vi "Disconnect.vi"(8 "error in (no error)":errorcluster, 11 "Network Stream in":refnum<class "Network Stream.lvclass">) -> (0 "error out":errorcluster, 3 "Network Stream out":refnum<class "Network Stream.lvclass">)   [LabVIEW 2020, in "Network Stream.lvclass"]
uses:
  Network Stream.lvclass
  Network Stream.lvclass/Network Stream.ctl
  <vilib>/dex/Flush And Wait Empty Condition.ctl
  <resource>/objmgr/ni.dex.rc
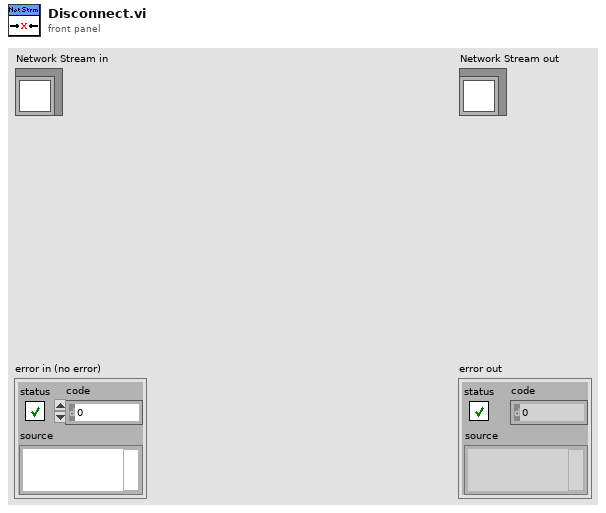
[diagram p1: front panel]
types:
  T1 = typedef "Flush And Wait Empty Condition.ctl" = u8
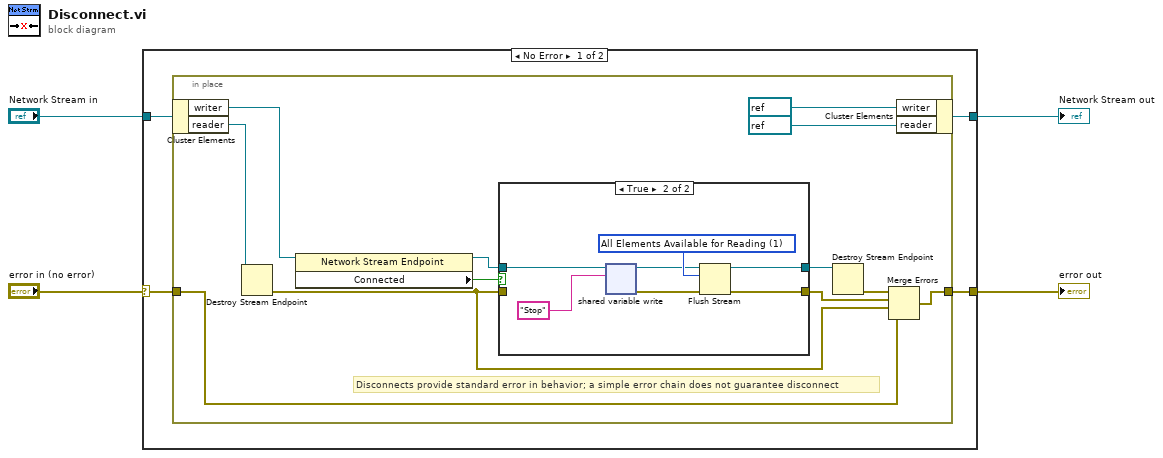
[diagram p0: block diagram]
diagram:
  n1 = case shown="No Error" "error in (no error)" {
    selector: "error in (no error)" -> [w8 w30]
    tunnel: [w5 w30] -> w1
    tunnel: [w7 w29] -> w3
    tunnel: "Network Stream in" -> [w6 w29]
    frame No Error {
      n2 = in-place {
        in-place-border: w8 -> [w9]
        in-place-border: [w12] -> w5
        # "Disconnects provide standard error in behavior; a simple error chain does not guarantee disconnect"
        n3 = in-place-cluster #1(w6) -> ("writer"=w19:refnum<k21>, "reader"=w13:refnum<k21>)
        n4 = Destroy Stream Endpoint(11:w13) -> (0:w10:errorcluster)  [unwired: 1 in]
        n5 = property class="Network Stream Endpoint"(reference=w19) -> (reference out=w18:refnum<k21>, "Connected"=w17:bool)  [unwired: 1 in, 1 out]
        n6 = case shown="True" w17 {
          tunnel: w10 -> [_ _]
          tunnel: [_ w27] -> w11
          tunnel: w18 -> [w21 w24]
          tunnel: [w21 w26] -> w14
          frame False {
          }
          frame True {
            w28 = T1 1 items=["All Elements Read From Stream", "All Elements Available for Reading"] ("wait condition")
            n7 = shared-variable-write(w24, "Stop" ("data in")) -> (w23:refnum<k21>, w25:errorcluster)  [unwired: 2 in, 1 out]
            n8 = Flush Stream(8:w25, 10:w28, 11:w23) -> (0:w27:errorcluster, 3:w26:refnum<k21>)  [unwired: 1 in, 1 out]
          }
        }
        n9 = Destroy Stream Endpoint(11:w14) -> (0:w15:errorcluster)  [unwired: 1 in]
        n10 = Merge Errors(w15, w11, w10, w9) -> (w12:errorcluster)
        n11 = in-place-cluster #1("writer"=refnum<k21> refnum, "reader"=refnum<k21> refnum) -> (w7:refnum<class "Network Stream.lvclass">)
      }
    }
    frame Error {
    }
  }
  "error out" <- w1
  "Network Stream out" <- w3
